vi "Prompt for Step.vi"(8 "error in (no error)":errorcluster, 10 "Subpanel Ref":refnum<vi>, 11 "Mouse Action in":refnum<class "Mouse Action.lvclass">) -> (0 "error out":errorcluster, 3 "Mouse Action out":refnum<class "Mouse Action.lvclass">)   [LabVIEW 2020, in "MacroAssert.lvlib" / "Mouse Action.lvclass"]
uses:
  Mouse Action.lvclass
  Mouse Action Type.ctl
  Action Step/Action Step.lvclass
panel:
  out "Subtype Description":string
  in  "Click Count":i32
  in  "Click Type":enum16{"Normal", "Hold", "Release"}(ring)
  in  "Y":i32
  in  "X":i32
  in  "Window/Control":string
  in  "Relative Type":T1(ring)
  in  "Button":enum16{"Left", "Right", "Middle"}(ring)
  in  "Delay":i32
  in  "Repeat":i32
  in  "Step Subtype":T2
  # "Left and right click at\nsame time to capture\ncurrent screen coords"
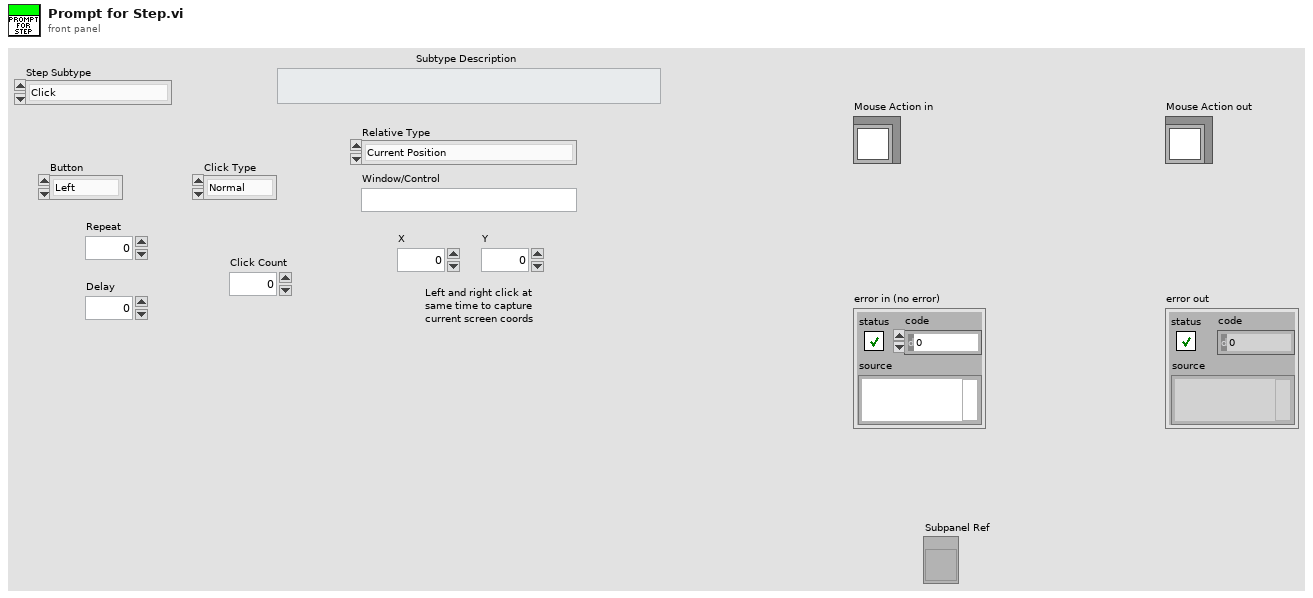
[diagram p1: front panel]
types:
  T1 = enum16{"Current Position", "Percentage of Screen", "Percentage from Top-Left of Control", "Pixels from Top-Left of Window", "Pixels from Top-Left of Control", "Percentage from Top-Left of Window"}
  T2 = typedef "MacroAssert.lvlib/Mouse Action.lvclass/Mouse Action Type.ctl" = enum16{"Click", "Absolute Move", "Absolute Move and Click", "Relative Move", "Relative Move and Click", "Wheel Up", "Wheel Down"}
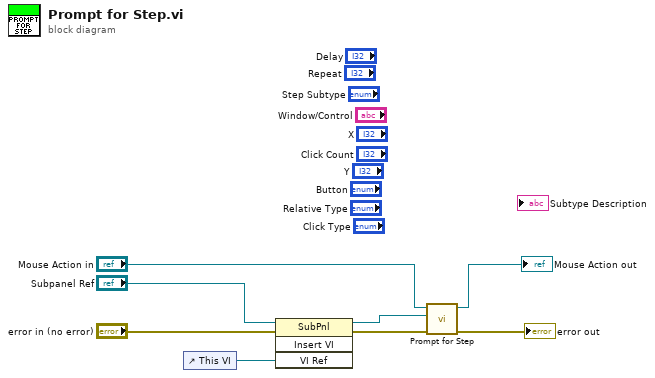
[diagram p0: block diagram]
diagram:
  n1 = control-ref of="This VI"() -> (w1:refnum<vi>)
  n2 = invoke class="SubPnl" method="Insert VI"(reference="Subpanel Ref", error in="error in (no error)", "VI Ref"=w1) -> (reference out=w2:refnum<vi>, error out=w4:errorcluster)  [unwired: 1 in, 2 out]
  n3 = call-parent "Prompt for Step.vi"("error in (no error)"=w4, "Subpanel Ref"=w2, "Step in"="Mouse Action in") -> ("error out"=→"error out":errorcluster, "Step out"=→"Mouse Action out":refnum<class "Mouse Action.lvclass">)  [unwired: 7 in]
